vi "Constants.vi"() -> ()   [LabVIEW 2020]
panel:
  in  "StartingPositionData":T1(array[cluster])=[{"Location"={"X"=0.0, "Y"=0.0}, "Angle"=0.0, "ReferencePoint"=enum."Center"}, {"Location"={"X"=289.5, "Y"=127.4}, "Angle"=65.0, "ReferencePoint"=enum."Center"}]
  in  "Track Width":dbl=23.4
  in  "CenterRotOffset":dbl=17.0
  in  "Length":dbl=39.0
  in  "Width":dbl=32.0
  # "LOCATIONS ARE 1 INDEXED!!!!! LOCATION 0 IS DEFAULT AND ALL 0's"
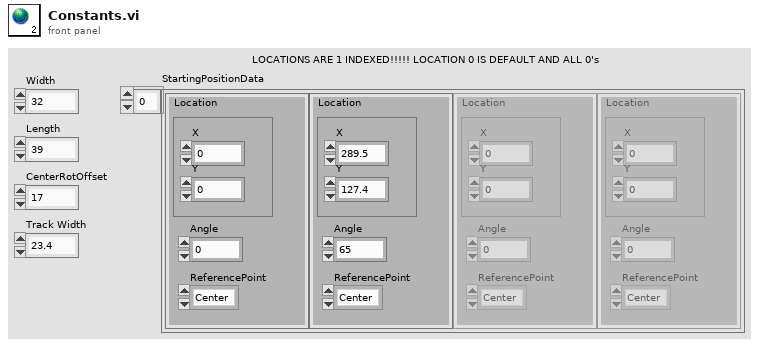
[diagram p1: front panel]
types:
  T1 = cluster{"Location":cluster{"X":dbl, "Y":dbl}, "Angle":dbl, "ReferencePoint":enum16{"Center", "FrontCenter", "FrontLeft", "FrontRight", "BackCenter", "BackLeft", "BackRight", "LeftCenter", "RightCenter"}}[]
diagram:
